vi "tm461_dcimgreader_wmetadata.vi"() -> ()   [LabVIEW 2023, in "HamamatsuCam.lvlib" / "HamamatsuCam.lvclass"]
uses:
  HamamatsuCam/HamamatsuCam/HamamatsuCam.lvclass
panel:
  out "Metadata Frame":string
  out "Metadata File":string
  out "Error Out":errorcluster
  out "Image":u16[][](graph)
  out "Time Stamp":dbl
  out "Total":i32
  in  "Index":i32 min=0 max=9 step=1
  out "Openfile":bool
  in  "Quit":bool
  in  "Open":bool
  in  "Frame Index":i32(c297)
  in  "DCIMG Path":path
  # "This is an example of how to read the images\nand metadata within a DCIMG file."
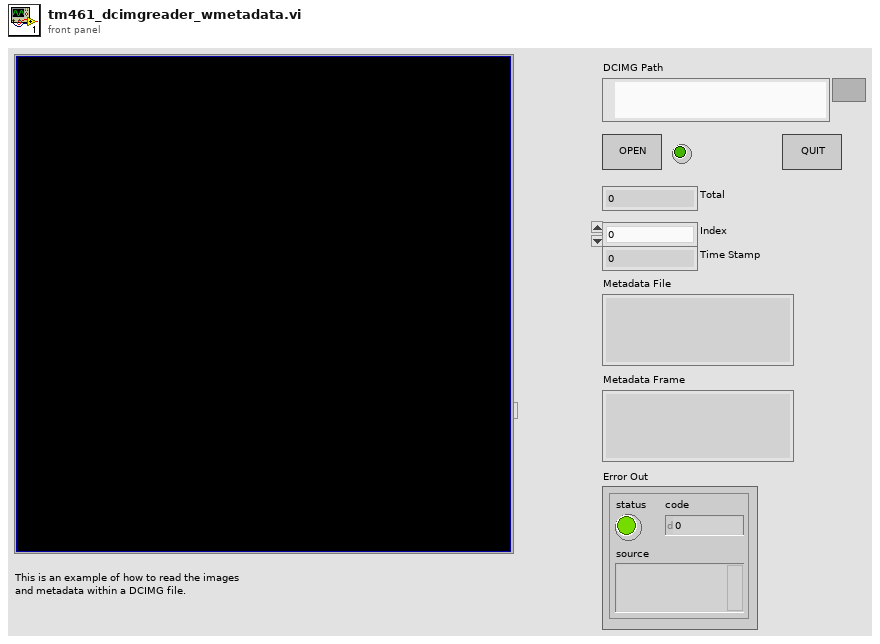
[diagram p1: front panel]
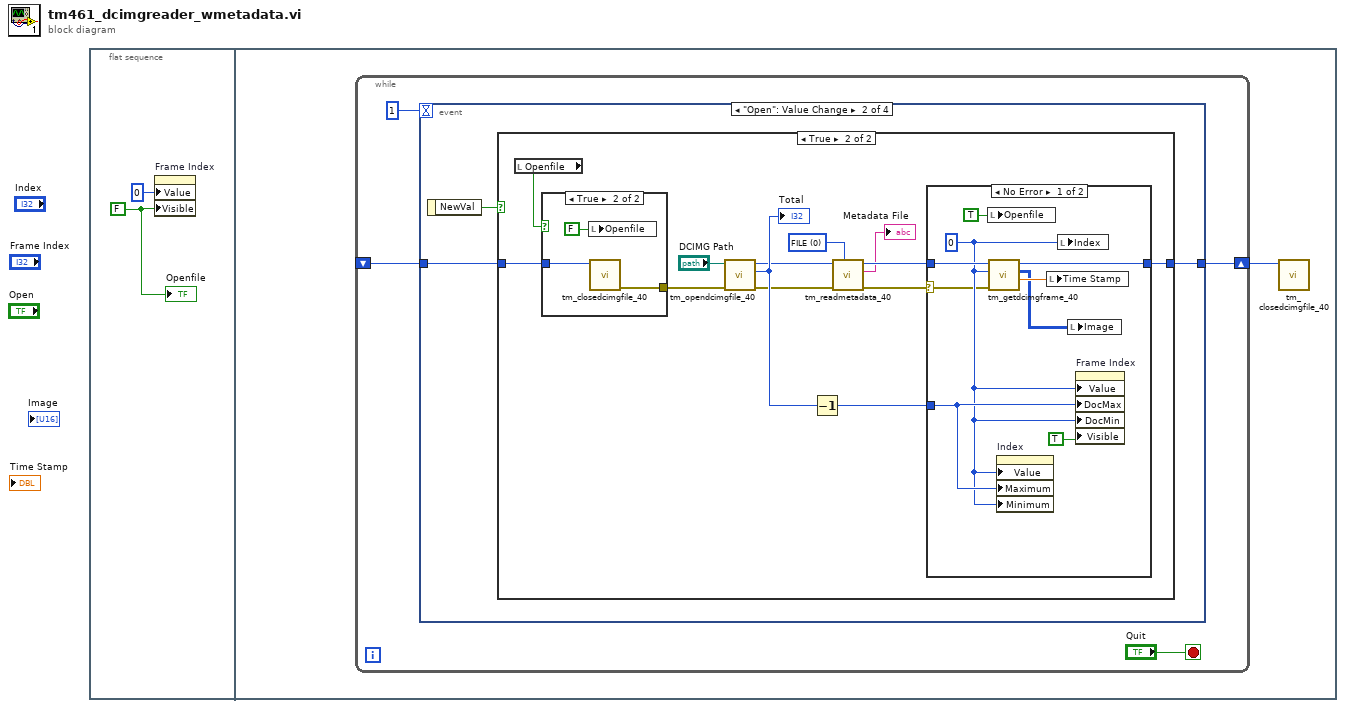
[diagram p0: block diagram]
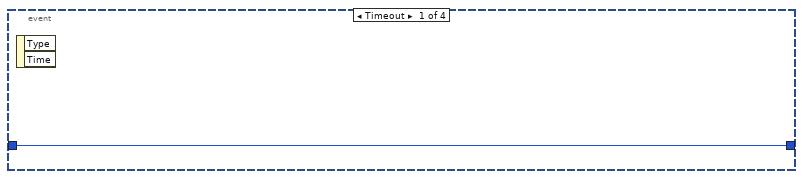
[diagram p2: hidden frame]
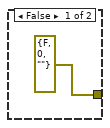
[diagram p4: hidden frame]
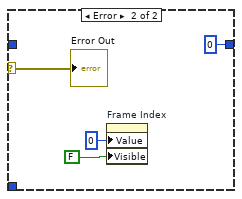
[diagram p5: hidden frame]
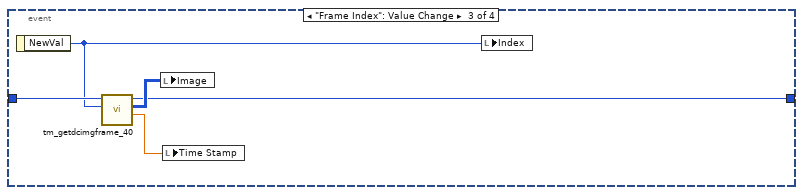
[diagram p6: hidden frame]
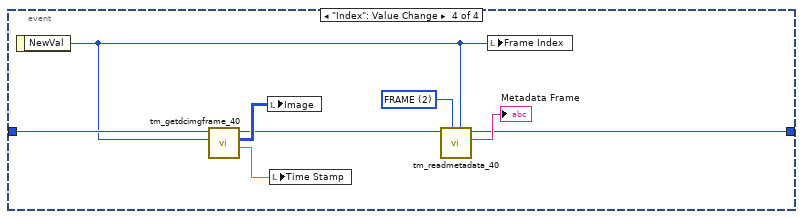
[diagram p7: hidden frame]
diagram:
  n1 = flat-sequence {
    frame #0 {
      w1 = FALSE ("Visible")
      n2 = property on="Frame Index" class="Scroll (strict)"("Value"=0 ("Frame Index"), "Visible"=w1) -> ()  [unwired: 2 in, 2 out]
      "Openfile" <- w1
    }
    frame #1 {
      n3 = while {
        shift-right: [w7] -> w3
        shift-left: _ -> [w6]
        stop <- "Quit" stop-if-true
        n4 = event shown="[1] \"Open\": Value Change" {
          selector: _ -> [_ _ _ _]
          dyn-events: _ -> [_ _ _ _]
          timeout: 1 -> [_ _ _ _]
          tunnel: [w8 w10 w43 w50] -> w7
          tunnel: w6 -> [w8 w9 w45 w55]
          event Timeout {
            n5 = event-data() -> ()  [unwired: 1 in, 2 out]
          }
          event "Open": Value Change {
            n6 = event-data() -> ("NewVal"=w11:bool)  [unwired: 1 in]
            n7 = case shown="True" w11 {
              tunnel: [w12 w25] -> w10
              tunnel: w9 -> [w12 w24]
              frame False {
              }
              frame True {
                w13 = 0 items=["FILE"=0, "FRAME"=2] ("Type")
                n8 = local read "Openfile"() -> (w23:bool)
                n9 = case shown="True" w23 {
                  tunnel: w24 -> [_ w29]
                  tunnel: [errorcluster {"status"=FALSE, "code"=0, "source"=""} ("error out") w27] -> w20
                  frame False {
                  }
                  frame True {
                    n10 = local write "Openfile"(FALSE ("Openfile")) -> ()
                    n11 = call "tm_closedcimgfile_40.vi"("File Handle"=w29) -> ("error out"=w27:errorcluster)  [unwired: 10 in]
                  }
                }
                n12 = call "tm_opendcimgfile_40.vi"("error in (no error)"=w20, "Path"="DCIMG Path") -> ("error out"=w17:errorcluster, "Total Frames"=w19:i32, "File Handle"=w18:u32)  [unwired: 7 in]
                "Total" <- w19
                n13 = Decrement(x=w19) -> (x-1=w22:i32)
                n14 = call "tm_readmetadata_40.vi"("Type"=w13, "error in (no error)"=w17, "File Handle"=w18) -> ("error out"=w15:errorcluster, "Metadata"=→"Metadata File":string, "File Handle"=w16:u32)  [unwired: 6 in]
                n15 = case shown="No Error" w15 {
                  selector: w15 -> [w31 w39]
                  tunnel: w16 -> [w38 _]
                  tunnel: w22 -> [w33 _]
                  tunnel: [w37 u32 0 ("File Handle out")] -> w25
                  frame No Error {
                    w32 = 0 ("Frame Index")
                    n16 = local write "Openfile"(TRUE ("Openfile")) -> ()
                    n17 = call "tm_getdcimgframe_40.vi"("error in (no error)"=w31, "Frame Index"=w32, "File Handle in"=w38) -> ("Timestamp"=w34:dbl, "Data"=w30:u16[][], "File Handle out"=w37:u32)  [unwired: 5 in, 1 out]
                    n18 = property on="Index" class="DigNum (strict)"("Value"=w32, "Maximum"=w33, "Minimum"=w32) -> ()  [unwired: 2 in, 2 out]
                    n19 = local write "Time Stamp"(w34) -> ()
                    n20 = local write "Index"(w32) -> ()
                    n21 = local write "Image"(w30) -> ()
                    n22 = property on="Frame Index" class="Scroll (strict)"("Value"=w32, "DocMax"=w33, "DocMin"=w32, "Visible"=TRUE) -> ()  [unwired: 2 in, 2 out]
                  }
                  frame Error {
                    n23 = property on="Frame Index" class="Scroll (strict)"("Value"=0 ("Frame Index"), "Visible"=FALSE) -> ()  [unwired: 2 in, 2 out]
                    "Error Out" <- w39
                  }
                }
              }
            }
          }
          event "Frame Index": Value Change {
            n24 = event-data() -> ("NewVal"=w44:i32)  [unwired: 1 in]
            n25 = call "tm_getdcimgframe_40.vi"("Frame Index"=w44, "File Handle in"=w45) -> ("Timestamp"=w46:dbl, "Data"=w47:u16[][], "File Handle out"=w43:u32)  [unwired: 6 in, 1 out]
            n26 = local write "Image"(w47) -> ()
            n27 = local write "Time Stamp"(w46) -> ()
            n28 = local write "Index"(w44) -> ()
          }
          event "Index": Value Change {
            w48 = 2 items=["FILE"=0, "FRAME"=2] ("Type")
            n29 = event-data() -> ("NewVal"=w49:i32)  [unwired: 1 in]
            n30 = call "tm_getdcimgframe_40.vi"("Frame Index"=w49, "File Handle in"=w55) -> ("Timestamp"=w53:dbl, "Data"=w54:u16[][], "File Handle out"=w51:u32)  [unwired: 6 in, 1 out]
            n31 = local write "Image"(w54) -> ()
            n32 = local write "Time Stamp"(w53) -> ()
            n33 = call "tm_readmetadata_40.vi"("Index"=w49, "Type"=w48, "File Handle"=w51) -> ("Metadata"=→"Metadata Frame":string, "File Handle"=w50:u32)  [unwired: 6 in, 1 out]
            n34 = local write "Frame Index"(w49) -> ()
          }
        }
      }
      n35 = call "tm_closedcimgfile_40.vi"("File Handle"=w3) -> ()  [unwired: 10 in, 1 out]
    }
  }
